vi "capex DC power.vi"() -> ()   [LabVIEW 2013]
panel:
  out "CV":bool
  out "CC":bool
  in  "DC Voltage":dbl
  in  "DC Amps":dbl
  in  "DC OVP":dbl
  in  "DC OCP":dbl
  out "DC volts":dbl
  out "DC amps":dbl
  out "OVP":dbl
  out "OCP":dbl
  in  "stop":bool
  in  "Enum":enum16{"2", "1"}(ring)
  in  "Command power supply":bool
  # "DC Volts"
  # "Amperes"
  # "Overvoltage protection limit"
  # "Overcurrent protection limit"
  # "Actual"
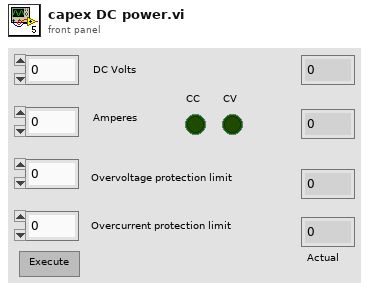
[diagram p1: front panel]
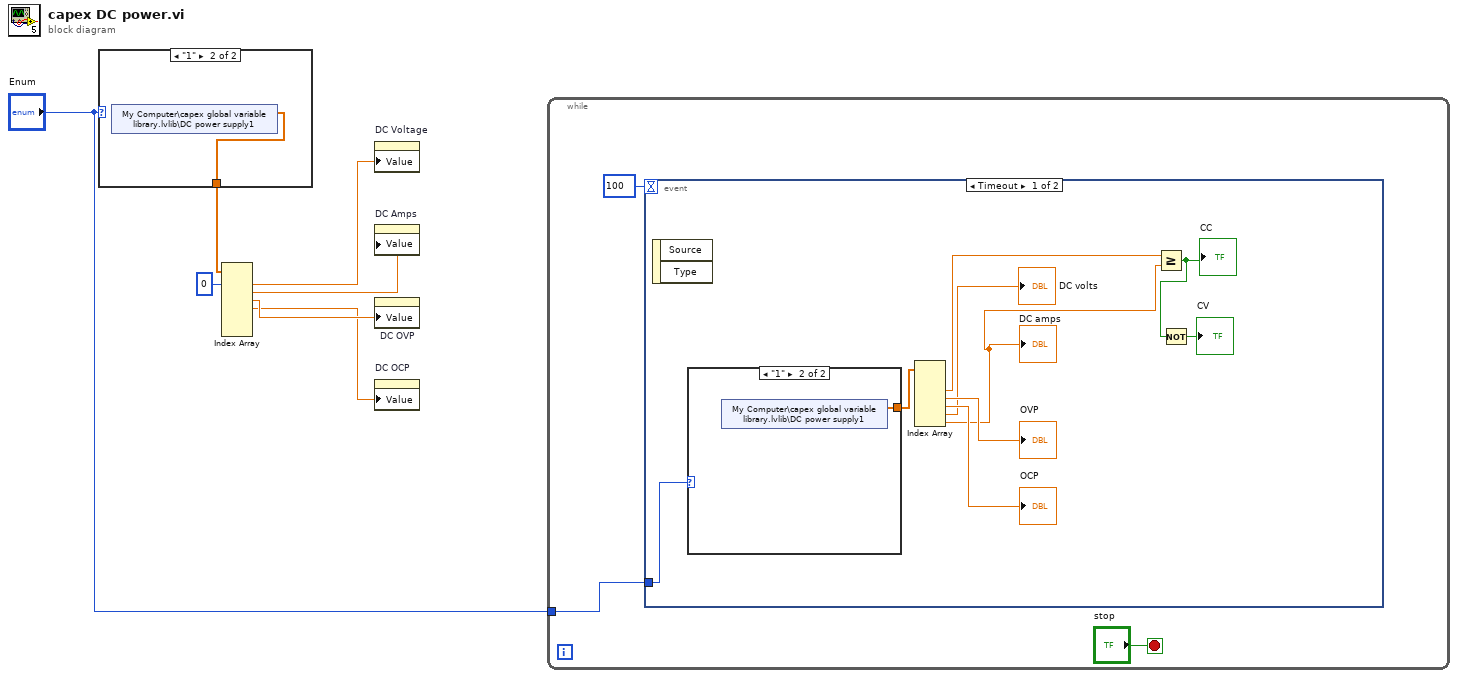
[diagram p0: block diagram]
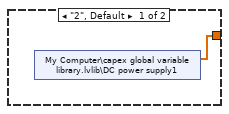
[diagram p2: hidden frame]
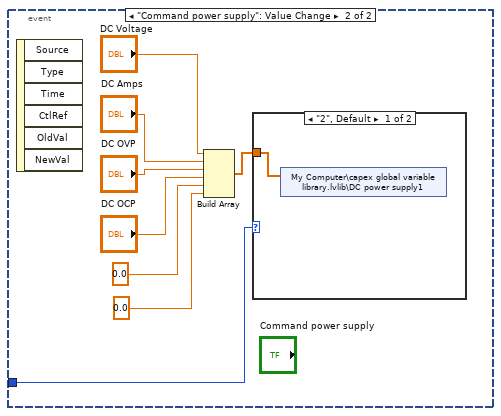
[diagram p3: hidden frame]
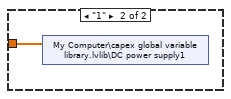
[diagram p4: hidden frame]
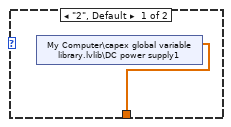
[diagram p5: hidden frame]
diagram:
  n1 = case shown="\"1\"" "Enum" {
    tunnel: [w8 w9] -> w2
    frame "2", Default {
      n2 = shared-variable "My Computer\\capex global variable library.lvlib\\DC power supply1"() -> (w8:dbl[])  [unwired: 1 in, 1 out]
    }
    frame "1" {
      n3 = shared-variable "My Computer\\capex global variable library.lvlib\\DC power supply1"() -> (w9:dbl[])  [unwired: 1 in, 1 out]
    }
  }
  n4 = Index Array(array=w2, index #1=0 ("index")) -> (element #1=w6:dbl, element #2=w5:dbl, element #3=w4:dbl, element #4=w3:dbl)  [unwired: 6 in, 3 out]
  n5 = property on="DC Voltage" class="DigNum (strict)"("Value"=w6) -> ()  [unwired: 2 in, 2 out]
  n6 = property on="DC Amps" class="DigNum (strict)"("Value"=w5) -> ()  [unwired: 2 in, 2 out]
  n7 = property on="DC OVP" class="DigNum (strict)"("Value"=w4) -> ()  [unwired: 2 in, 2 out]
  n8 = property on="DC OCP" class="DigNum (strict)"("Value"=w3) -> ()  [unwired: 2 in, 2 out]
  n9 = while {
    tunnel: "Enum" -> [w12]
    stop <- "stop" stop-if-true
    n10 = event shown="[0] Timeout" {
      selector: _ -> [_ _]
      dyn-events: _ -> [_ _]
      timeout: 100 -> [_ _]
      tunnel: w12 -> [w21 w24]
      event Timeout {
        n11 = event-data() -> ()  [unwired: 1 in, 2 out]
        n12 = case shown="\"1\"" w21 {
          tunnel: [w22 w23] -> w20
          frame "2", Default {
            n13 = shared-variable "My Computer\\capex global variable library.lvlib\\DC power supply1"() -> (w22:dbl[])  [unwired: 1 in, 1 out]
          }
          frame "1" {
            n14 = shared-variable "My Computer\\capex global variable library.lvlib\\DC power supply1"() -> (w23:dbl[])  [unwired: 1 in, 1 out]
          }
        }
        n15 = Index Array(array=w20) -> (element #2=w17:dbl, element #3=→"OVP":dbl, element #4=→"OCP":dbl, element #5=→"DC volts":dbl, element #6=w15:dbl)  [unwired: 6 in, 1 out]
        "DC amps" <- w15
        n16 = Greater Or Equal?(x=w17, y=w15) -> (x >= y?=w13:bool)
        "CC" <- w13
        n17 = Not(x=w13) -> (.not. x?=→"CV":bool)
      }
      event "Command power supply": Value Change {
        n18 = event-data() -> ()  [unwired: 1 in, 6 out]
        n19 = Build Array("DC Voltage", "DC Amps", "DC OVP", "DC OCP", 0.0 ("element"), 0.0 ("element")) -> (w27:dbl[])
        n20 = case shown="\"2\", Default" w24 {
          tunnel: w27 -> [w32 w33]
          frame "2", Default {
            n21 = shared-variable "My Computer\\capex global variable library.lvlib\\DC power supply1"(w32) -> ()  [unwired: 1 in, 1 out]
          }
          frame "1" {
            n22 = shared-variable "My Computer\\capex global variable library.lvlib\\DC power supply1"(w33) -> ()  [unwired: 1 in, 1 out]
          }
        }
      }
    }
  }
